vi "string to boolean array.vi"(4 "String Input":string) -> (1 "Boolean array":bool[](array[boolean]))   [LabVIEW 2020]
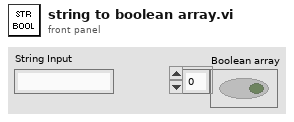
[diagram p1: front panel]
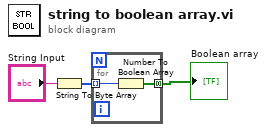
[diagram p0: block diagram]
diagram:
  n1 = String To Byte Array(string="String Input") -> (unsigned byte array=w3:u8[])
  n2 = for {
    tunnel: w3 -> [w5] mode=indexing
    tunnel: [w4] -> w1 mode=concatenating
    n3 = Number To Boolean Array(number=w5) -> (Boolean array=w4:bool[])
  }
  "Boolean array" <- w1
